vi "Control Gas Heater.vi"(0 "Session Handle in":T1, 7 "On?":bool=TRUE, 11 "error in (no error)":errorcluster) -> (4 "Session Handle out":T1, 6 "Success?":bool, 15 "error out":errorcluster)   [LabVIEW 2015, in "Gas.lvclass"]
uses:
  Gas.lvclass
  Typedefs/Session Handle.ctl
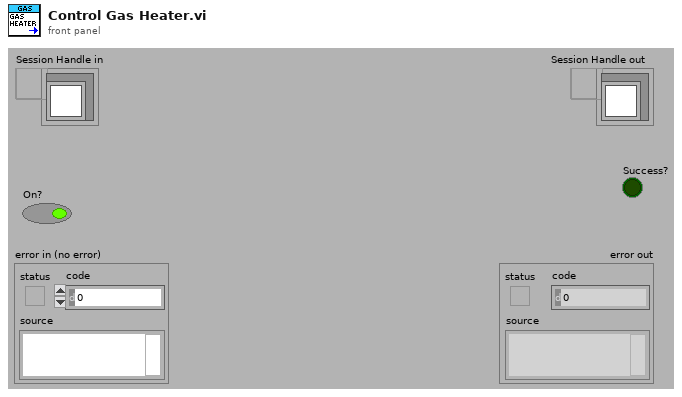
[diagram p1: front panel]
types:
  T1 = typedef "Gas.lvclass/Session Handle.ctl" = refnum<data-value>
  T2 = typedef "XNET Frame CAN.ctl" = cluster{"timestamp":timestamp, "payload":u8[], "identifier":u32, "type":T3, "extended?":bool, "echo?":bool}
  T3 = typedef "XNET Frame Type CAN.ctl" = u8
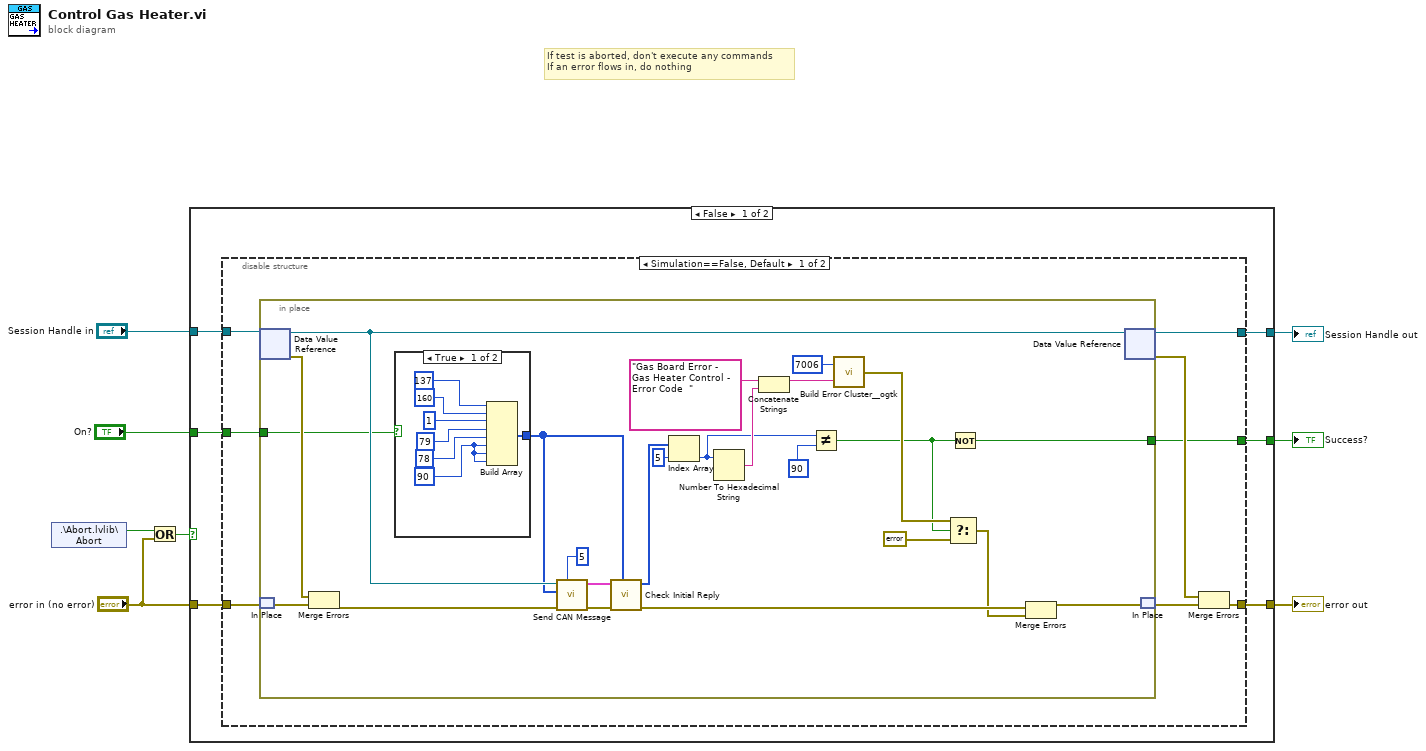
[diagram p0: block diagram]
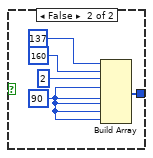
[diagram p2: hidden frame]
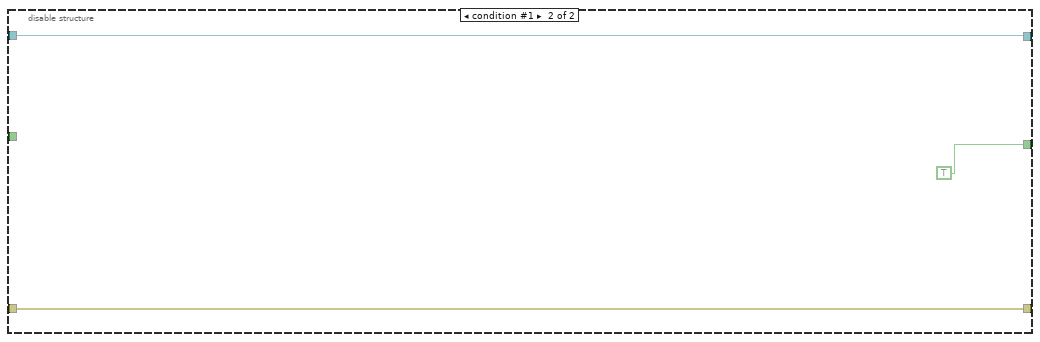
[diagram p3: hidden frame]
diagram:
  # "If test is aborted, don't execute any commands\nIf an error flows in, do nothing"
  n1 = shared-variable ".\\Abort.lvlib\\Abort"() -> (w5:bool)  [unwired: 1 in, 1 out]
  n2 = Or(x=w5, y="error in (no error)") -> (x .or. y?=w3:bool)
  n3 = case shown="False" w3 {
    tunnel: [w14 w63] -> w7
    tunnel: [w13 w62] -> w6
    tunnel: "Session Handle in" -> [w12 w63]
    tunnel: "error in (no error)" -> [w11 w62]
    tunnel: [w10 _] -> w2
    tunnel: "On?" -> [w9 _]
    frame False {
      n4 = disable-structure shown="Simulation==False, Default" {
        disable-tunnel: [w22 w61] -> w14
        disable-tunnel: [w19 w60] -> w13
        disable-tunnel: w12 -> [w18 w61]
        disable-tunnel: w11 -> [w17 w60]
        disable-tunnel: [w16 TRUE] -> w10
        disable-tunnel: w9 -> [w15 _]
        frame condition #0 (active) {
          n5 = in-place {
            in-place-border: [w36] -> w16
            in-place-border: w15 -> [w35]
            n6 = in-place-dvr #1(w18) -> (w42:refnum<class "Gas.lvclass">, w45:errorcluster)
            n7 = in-place-match #2(w17) -> (w44:errorcluster)
            n8 = Merge Errors(w45, w44) -> (w43:errorcluster)
            n9 = case shown="True" w35 {
              tunnel: [w49 w56] -> w34
              frame True {
                w48 = u8 90 ("new element/subarray")
                n10 = Build Array(u8 137 ("new element/subarray"), u8 160 ("new element/subarray"), u8 1 ("new element/subarray"), u8 79 ("new element/subarray"), u8 78 ("new element/subarray"), w48, w48, w48) -> (w49:u8[])
              }
              frame False {
                w54 = u8 90 ("new element/subarray")
                n11 = Build Array(u8 137 ("new element/subarray"), u8 160 ("new element/subarray"), u8 2 ("new element/subarray"), w54, w54, w54, w54, w54) -> (w56:u8[])
              }
            }
            n12 = call "Send CAN Message.vi"("Number of Retries"=5, "error in (no error)"=w43, "payload"=w34, "Gas In"=w42) -> ("error out"=w25:errorcluster, "Reply"=w40:T2[])  [unwired: 5 in, 1 out]
            n13 = call "Check Initial Reply.vi"("Write Message"=w34, "error in (no error)"=w25, "Reply"=w40) -> ("error out"=w24:errorcluster, "Data Packet"=w33:u8[])  [unwired: 5 in, 2 out]
            n14 = Index Array(array=w33, index=5) -> (element=w28:u8)
            n15 = Number To Hexadecimal String(2:w28) -> (0:w30:string)  [unwired: 1 in]
            n16 = Concatenate Strings("Gas Board Error -  Gas Heater Control - Error Code  " ("string"), w30) -> (w29:string)
            n17 = Not Equal?(x=w28, y=u8 90 ("new element/subarray")) -> (x != y?=w26:bool)
            n18 = call <userlib>:"Build Error Cluster__ogtk.vi"("String to Prepend to source (\"\")"=w29, "code"=7006) -> ("error out"=w38:errorcluster)
            n19 = Select(t=w38, s=w26, f=errorcluster {"status"=FALSE, "code"=0, "source"=""}) -> (s? t:f=w23:errorcluster)
            n20 = Not(x=w26) -> (.not. x?=w36:bool)
            n21 = Merge Errors(w24, w23) -> (w46:errorcluster)
            n22 = in-place-dvr #1(w42) -> (w22:T1, w20:errorcluster)
            n23 = in-place-match #2(w46) -> (w21:errorcluster)
          }
          n24 = Merge Errors(w20, w21) -> (w19:errorcluster)
        }
        frame condition #1 {
        }
      }
    }
    frame True {
    }
  }
  "Session Handle out" <- w7
  "error out" <- w6
  "Success?" <- w2
